vi "Exp3.vi"() -> ()   [LabVIEW 2018]
uses:
  <vilib>/Platform/TimedLoop/XDataNode/timing_clust.ctl
  <vilib>/Platform/TimedLoop/XDataNode/nitl_modes.ctl
  <vilib>/Platform/TimedLoop/XDataNode/wakeup.ctl
  <vilib>/MakerHub/LINX/Public/Peripherals/Analog/Analog Read 1 Chan.vi
  <vilib>/MakerHub/LINX/Public/Peripherals/PWM/PWM Set Duty Cycle 1 Chan.vi
  <vilib>/MakerHub/LINX/Public/Peripherals/Analog/Analog Read N Chans.vi
  <vilib>/MakerHub/LINX/Private/Local IO/LinxAnalogRead.vi
  <vilib>/MakerHub/LINX/Public/Utilities/Check Channel.vi
  <vilib>/MakerHub/LINX/Public/Utilities/Open Serial.vi
  <vilib>/MakerHub/LINX/Private/Utilties/Generate Error.vi
  <vilib>/MakerHub/LINX/Public/Peripherals/PWM/PWM Set Duty Cycle N Chans.vi
  <vilib>/platform/TimedLoop/XDataNode/XDataNode.xnode
  <vilib>/MakerHub/LINX/LMH-LINX.lvlib
  <vilib>/Platform/TimedLoop/XDataNode/XDNodeRunTimeDep.lvlib
panel:
  out "T0":dbl
  in  "Tab Control":enum32{"Monitoring", "TDTC Model"}(tab)
  in  "Serial Port":refnum<visa-resource-name>="COM4"
  out "Period":i64
  in  "T_des":dbl=50.0
  in  "Kp":dbl=50.0
  out "Temperature":cluster{dbl, "output":dbl}(graph)={31.0, "output"=73.73046875}
  in  "Smith predictor":bool=TRUE
  in  "Kss":dbl=1.1
  in  "Theta":dbl=9.49
  in  "Tau":dbl=232.06
  in  "Stop Button":bool
  # "Room temperature"
  # "TDTC Model Parameters"
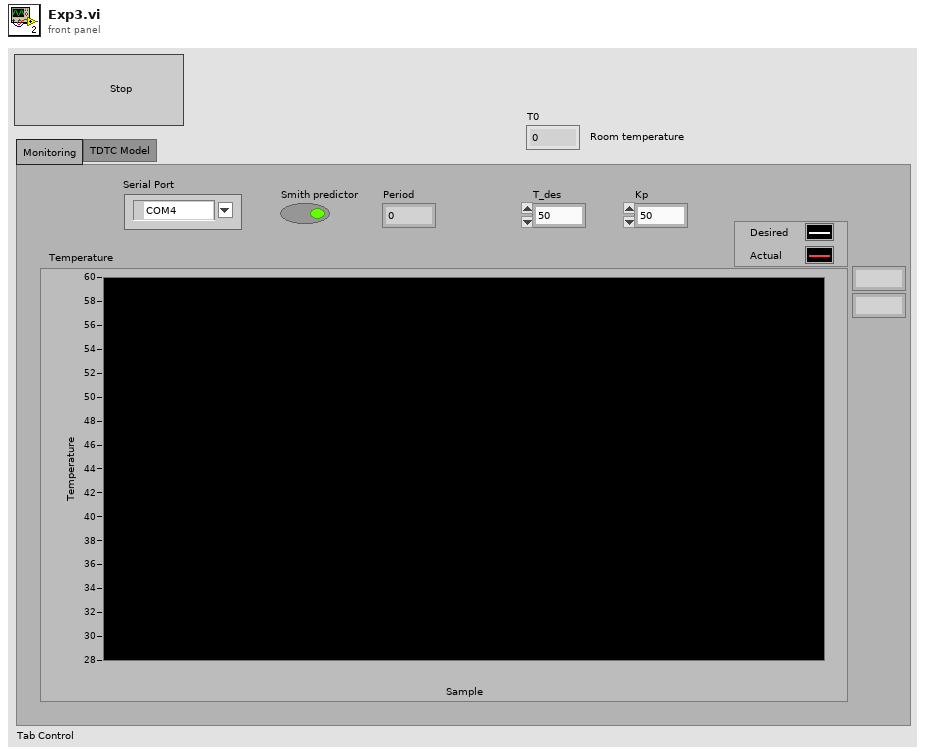
[diagram p1: front panel]
types:
  T1 = enum16{"open", "replace", "create", "open or create", "replace or create", "replace or create with confirmation"}
  T2 = typedef "XDNodeRunTimeDep.lvlib/timing_clust.ctl" = cluster{"Expected End [f-1]":u64, "Actual End [f-1]":u64, "Finished Late? [f-1]":bool, "Expected End [i-1]":u64, "Actual End [i-1]":u64, "Finished Late? [i-1]":bool, "Expected Start [i]":u64, "Actual Start [i]":u64, "Expected Start [f]":u64, "Actual Start [f]":u64, "Source Name":string, "Structure Name":string, "Period":i64, "Deadline":i64, "Offset":i64, "Start":i64, "Priority":i32, "Timeout":i32, "Mode":T3, "Wakeup Reason":T4, "Error":errorcluster, "Source Type":string, "Secondary Source Type":string, "Global End Time":u64, "Global Start Time":u64, "Frame Duration":u64, "Iteration Duration":u64, "Assigned CPU":i32, "I/O Scan Engine Mode":u32}
  T3 = typedef "XDNodeRunTimeDep.lvlib/nitl_modes.ctl" = enum32{"No Change", "Process missed periods, maintain original phase", "Discard missed periods, maintain original phase", "Process missed periods, ignore original phase", "Discard missed periods, ignore original phase"}
  T4 = typedef "XDNodeRunTimeDep.lvlib/wakeup.ctl" = enum32{"Normal", "Aborted", "Asynchronous wakeup", "Timing source error", "Timed loop error", "Timeout"}
  T5 = typedef "LMH-LINX.lvlib/LINX Ref.ctl" = cluster{"IO":T6, "Interface":T7, "LINX Device Config":T8}
  T6 = typedef "LMH-LINX.lvlib/Platform.ctl" = enum16{"Remote", "Local"}
  T7 = typedef "LMH-LINX.lvlib/Interface.ctl" = enum16{"Serial", "TCP"}
  T8 = typedef "LMH-LINX.lvlib/Device.lvlib/LINX Device Config.ctl" = cluster{"Interface":T7, "COM Port":refnum<visa-resource-name>, "TCP Configuration":T9, "Device Family":u8, "Device ID":u8, "Device Name":string, "TCP Ref":refnum<k5>, "Channels":T10}
  T9 = typedef "LMH-LINX.lvlib/Device.lvlib/TCP Config.ctl" = cluster{"IP Address":string, "Port":u16}
  T10 = typedef "LMH-LINX.lvlib/Channels.ctl" = cluster{"DI":u8[], "DO":u8[], "AI":u8[], "AO":u8[], "PWM":u8[], "QE":u8[], "UART":u8[], "I2C 2":u8[], "SPI":u8[], "CAN":u8[], "Servo":u8[], "AI Ref (V)":dbl, "AI Resolution (Bits)":u8, "AO Ref (V)":dbl, "AO Resolution (Bits)":u8}
  T11 = enum16{"big-endian, network order", "native, host order", "little-endian"}
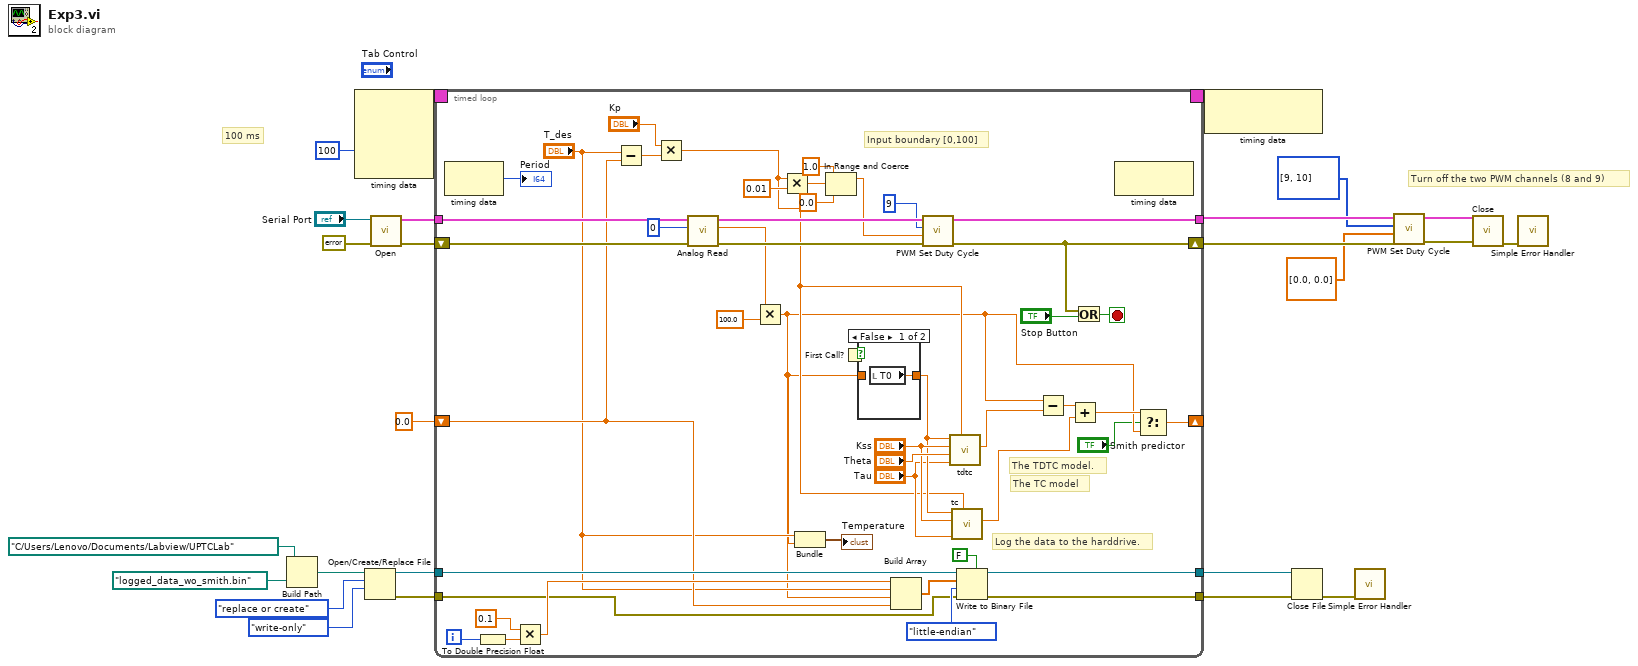
[diagram p0: block diagram]
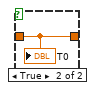
[diagram p2: hidden frame]
diagram:
  # "100 ms"
  # "Turn off the two PWM channels (8 and 9)"
  n1 = Build Path(base path=path "C:/Users/Lenovo/Documents/Labview/UPTCLab", name or relative path=path "logged_data_wo_smith.bin" ("default name")) -> (appended path=w4:path)
  n2 = node-c288(i64 100 ("Period")) -> (w20:T2)  [unwired: 3 in]
  n3 = Open/Create/Replace File(file path (use dialog)=w4, operation (0:open)=T1."replace or create", access (0:read/write)=enum16{"read/write", "read-only", "write-only"}."write-only") -> (refnum out=w8:refnum<file>, error out=w2:errorcluster)  [unwired: 3 in, 1 out]
  n4 = call-poly <vilib>:"Open.vi"("Error In"=errorcluster {"status"=FALSE, "code"=0, "source"=""}, "Serial Port"="Serial Port") -> ("Error Out"=w24:errorcluster, "LINX Resource"=w25:T5)  [unwired: 7 in, 1 out]
  n5 = timed-loop {
    tunnel: w25 -> [w70]
    tunnel: [w65] -> w16
    shift-right: [w64] -> w15
    shift-left: w24 -> [w69]
    timing: w20 -> [_]
    timing-out: [_] -> w19
    tunnel: w8 -> [w54]
    tunnel: [w47] -> w6
    tunnel: [w46] -> w5
    tunnel: w2 -> [w42]
    shift-right: [w27] -> _
    shift-left: 0.0 -> [w32]
    i -> [w53]
    stop <- w72 stop-if-true
    # "The TC model"
    # "Log the data to the harddrive."
    # "The TDTC model."
    # "Input boundary [0,100]"
    n6 = node-c288() -> (→"Period":i64)  [unwired: 1 in]
    n7 = To Double Precision Float(number=w53) -> (double precision float=w52:dbl)
    n8 = Multiply(x=0.1, y=w52) -> (x*y=w45:dbl)
    n9 = Subtract(x="T_des", y=w32) -> (x-y=w35:dbl)
    n10 = Multiply(x="Kp", y=w35) -> (x*y=w33:dbl)
    n11 = call-poly <vilib>:"Analog Read.vi"("Error In"=w69, "Analog Channel"=u8 0, "LINX Resource"=w70) -> ("Error Out"=w66:errorcluster, "Voltage"=w62:dbl, "LINX Resource"=w67:T5)  [unwired: 5 in, 1 out]
    n12 = Multiply(x=w62, y=100.0) -> (x*y=w28:dbl)
    n13 = Multiply(x=w33, y=0.01) -> (x*y=w58:dbl)
    n14 = Bundle("T_des"="T_des", w28) -> (→"Temperature":cluster{"T_des":dbl, dbl})  [unwired: 1 in]
    n15 = In Range and Coerce(upper limit=1.0, x=w58, lower limit=0.0) -> (coerced(x)=w57:dbl)  [unwired: 1 out]
    n16 = First Call?() -> (First Call?: T/F=w43:bool)
    n17 = case shown="False" w43 {
      tunnel: w28 -> [_ w74]
      tunnel: [w73 w74] -> w40
      frame False {
        n18 = local read "T0"() -> (w73:dbl)
      }
      frame True {
        "T0" <- w74
      }
    }
    n19 = Build Array(w45, "T_des", w28, w32) -> (w50:dbl[])
    n20 = call-poly <vilib>:"PWM Set Duty Cycle.vi"("Error In"=w66, "Duty Cycle (0-1)"=w57, "PWM Channel"=u8 9, "LINX Resource"=w67) -> ("Error Out"=w64:errorcluster, "LINX Resource"=w65:T5)  [unwired: 6 in]
    n21 = call "tdtc.vi"("input"=w33, "Tau"="Tau", "Theta"="Theta", "Kss"="Kss", "T0"=w40) -> ("output"=w38:dbl)  [unwired: 6 in]
    n22 = call "tc.vi"("input"=w33, "Tau"="Tau", "Kss"="Kss", "T0"=w40) -> ("output"=w36:dbl)  [unwired: 7 in]
    n23 = Write to Binary File(file (use dialog)=w54, data=w50, error in=w42, 5:FALSE ("prepend array or string size? (T)"), 9:T11."little-endian" ("byte order (0:big-endian, network order)")) -> (refnum out=w47:refnum<file>, error out=w46:errorcluster)  [unwired: 1 in, 1 out]
    n24 = Subtract(x=w28, y=w38) -> (x-y=w37:dbl)
    n25 = Add(x=w37, y=w36) -> (x+y=w29:dbl)
    n26 = Or(x=w64, y="Stop Button") -> (x .or. y?=w72:bool)
    n27 = node-c288() -> ()  [unwired: 1 in, 1 out]
    n28 = Select(t=w29, s="Smith predictor", f=w28) -> (s? t:f=w27:dbl)
  }
  n29 = node-c288(w19) -> ()  [unwired: 1 out]
  n30 = Close File(refnum=w6, error in=w5) -> (error out=w7:errorcluster)  [unwired: 1 out]
  n31 = call <vilib>:"Simple Error Handler.vi"("error in (no error)"=w7) -> ()  [unwired: 4 in, 5 out]
  n32 = call-poly <vilib>:"PWM Set Duty Cycle.vi"("Error In"=w15, "Duty Cycles"=dbl[] [0.0, 0.0], "PWM Channels"=u8[] [9, 10], "LINX Resource"=w16) -> ("Error Out"=w14:errorcluster, "LINX Resource"=w17:T5)  [unwired: 6 in]
  n33 = call <vilib>:"Close.vi"("Error In"=w14, "LINX Resource"=w17) -> ("Error Out"=w22:errorcluster)  [unwired: 9 in]
  n34 = call <vilib>:"Simple Error Handler.vi"("error in (no error)"=w22) -> ()  [unwired: 4 in, 5 out]
